vi "河内塔-全塔绘图.vi"(4 "N":u8, 8 "绘图区域大小":cluster{"Width":u32, "Height":u32}, 9 "C":u8[](array[numeric]), 10 "B":u8[](array[numeric]), 11 "A":i32[](array[numeric])) -> (3 "新图片":picture)   [LabVIEW 2016]
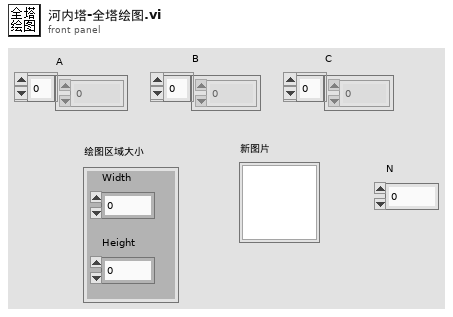
[diagram p1: front panel]
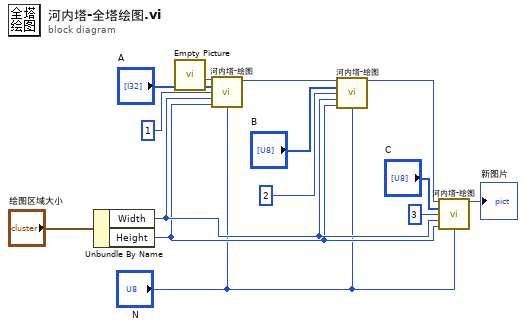
[diagram p0: block diagram]
diagram:
  n1 = Unbundle By Name("绘图区域大小") -> ("Width"=w4:u32, "Height"=w2:u32)
  n2 = call "Empty Picture"() -> ("empty picture"=w5:picture)
  n3 = call "河内塔-绘图.vi"("图片"=w5, "Value"="A", "第几塔"=1, "Width"=w4, "Height"=w2, "N"="N") -> ("新图片"=w10:picture)  [unwired: 9 in]
  n4 = call "河内塔-绘图.vi"("图片"=w10, "Value"="B", "第几塔"=2, "Width"=w4, "Height"=w2, "N"="N") -> ("新图片"=w11:picture)  [unwired: 9 in]
  n5 = call "河内塔-绘图.vi"("图片"=w11, "Value"="C", "第几塔"=3, "Width"=w4, "Height"=w2, "N"="N") -> ("新图片"=→"新图片":picture)  [unwired: 9 in]
